vi "Untitled 2.vi"() -> ()   [LabVIEW 2013]
uses:
  cal_p.vi
panel:
  out "Waveform Graph":dbl[](graph)
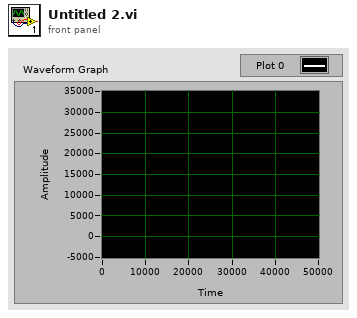
[diagram p1: front panel]
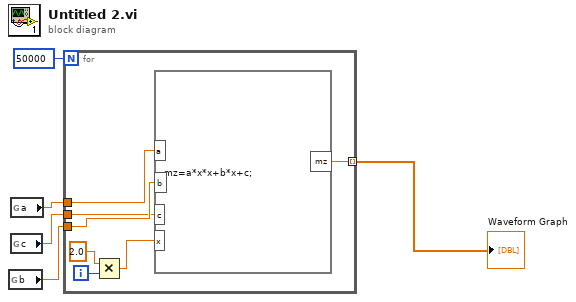
[diagram p0: block diagram]
diagram:
  n1 = global read "cal_p.vi" "b"() -> (w4:dbl)
  n2 = global read "cal_p.vi" "a"() -> (w5:dbl)
  n3 = global read "cal_p.vi" "c"() -> (w3:dbl)
  n4 = for {
    N: 50000 -> [_]
    tunnel: [w12] -> w1 mode=indexing
    tunnel: w3 -> [w9]
    tunnel: w4 -> [w10]
    tunnel: w5 -> [w11]
    i -> [w8]
    n5 = Multiply(x=2.0, y=w8) -> (x*y=w6:dbl)
    n6 = formula code="mz=a*x*x+b*x+c;"("a"=w11, "b"=w10, "c"=w9, "x"=w6) -> ("mz"=w12:dbl)
  }
  "Waveform Graph" <- w1
